vi "DS1820TEMP 3.vi"() -> ()   [LabVIEW 2017]
uses:
  <vilib>/Instr/_visa.llb/VISA Configure Serial Port (Instr).vi
panel:
  in  "stop":bool
  in  "Lim_inf":dbl
  in  "Lim_sup":dbl
  out "WAVE TEMP":dbl(graph)
  out "TEMP GAUGE":dbl(slide) scale=0.0..100.0
  out "TEMP":string
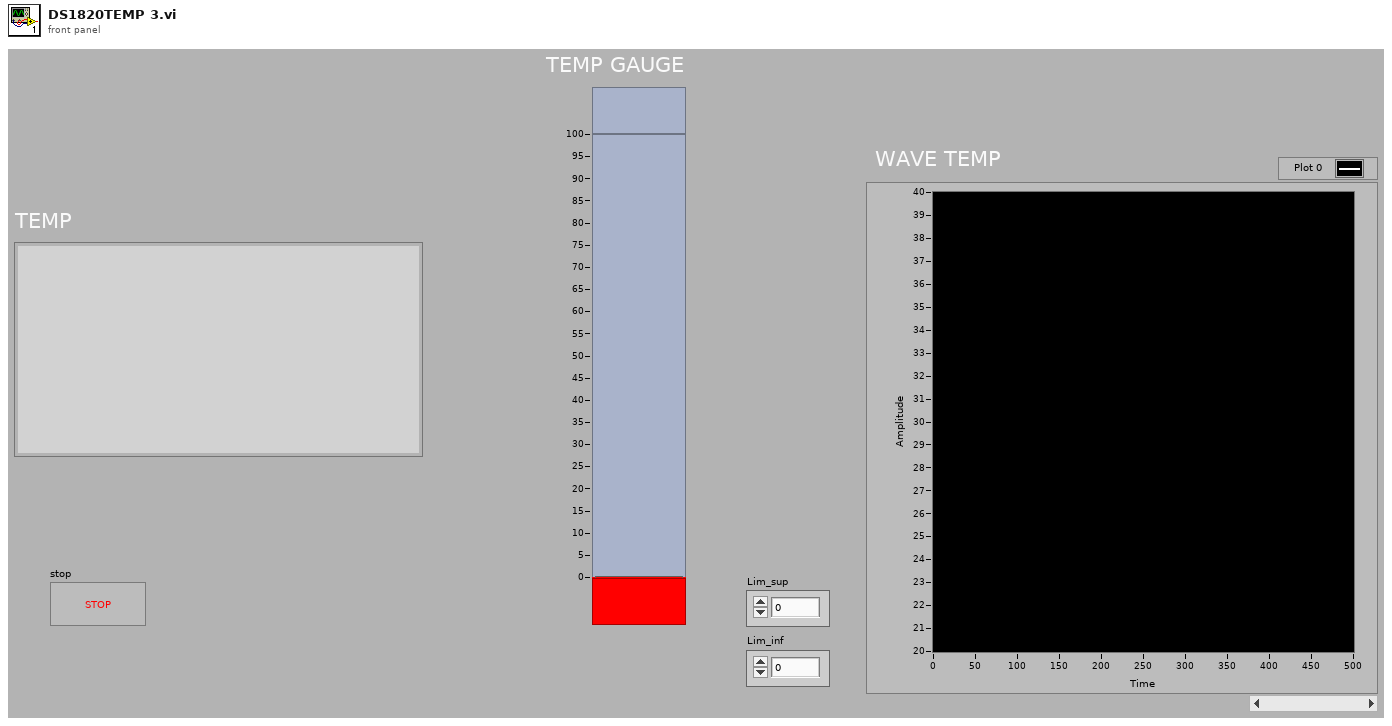
[diagram p1: front panel]
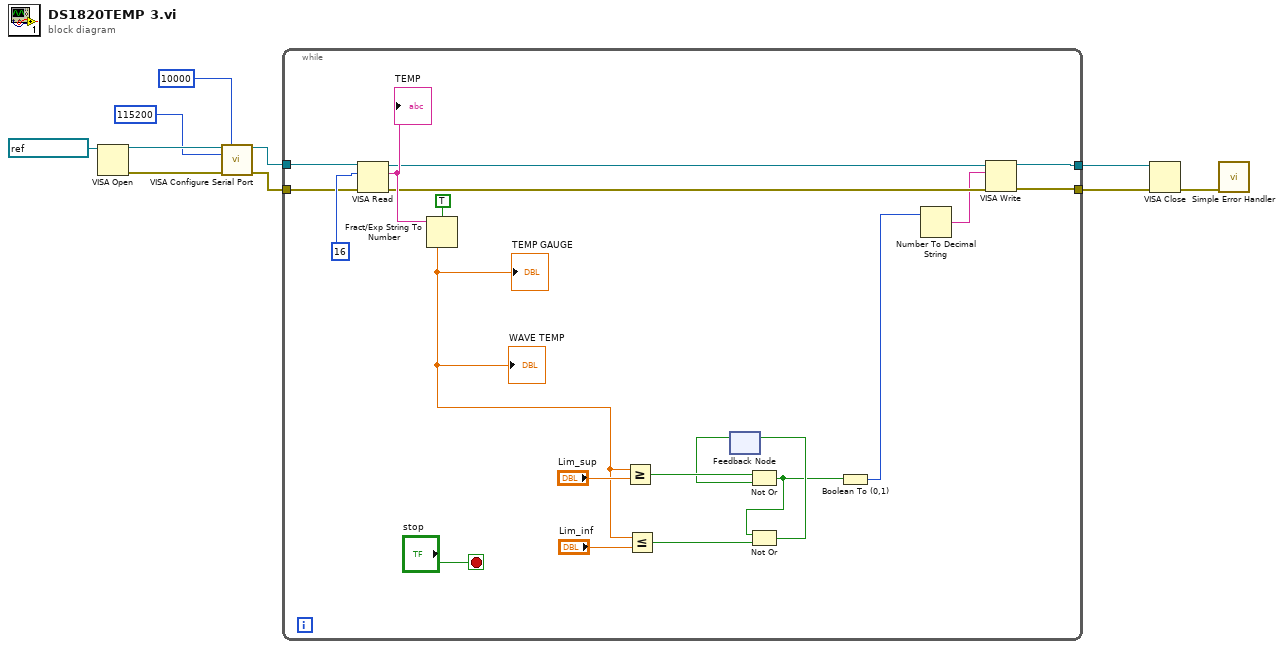
[diagram p0: block diagram]
diagram:
  n1 = VISA Open(VISA resource name=refnum<visa-resource-name> "COM3") -> (VISA resource name=w6:refnum<visa-resource-name>, error out=w5:errorcluster)  [unwired: 4 in]
  n2 = call-poly "VISA Configure Serial Port"("VISA resource name"=w6, "timeout (10sec)"=u32 10000, "baud rate (9600)"=u32 115200, "error in (no error)"=w5) -> ("VISA resource name out"=w8:refnum<visa-resource-name>, "error out"=w7:errorcluster)  [unwired: 10 in]
  n3 = while {
    tunnel: [w15] -> w10
    tunnel: [w14] -> w9
    tunnel: w8 -> [w19]
    tunnel: w7 -> [w18]
    stop <- "stop" stop-if-true
    n4 = VISA Read(VISA resource name=w19, byte count=u32 16, error in (no error)=w18) -> (VISA resource name out=w17:refnum<visa-resource-name>, read buffer=w30:string, error out=w16:errorcluster)  [unwired: 1 out]
    "TEMP" <- w30
    n5 = Fract/Exp String To Number(use system decimal point (T)=TRUE, string=w30) -> (number=w22:dbl)  [unwired: 2 in, 1 out]
    "TEMP GAUGE" <- w22
    "WAVE TEMP" <- w22
    n6 = Greater Or Equal?(x=w22, y="Lim_sup") -> (x >= y?=w27:bool)
    n7 = Less Or Equal?(x=w22, y="Lim_inf") -> (x <= y?=w28:bool)
    n8 = feedback #1() -> (w26:bool)  [unwired: 1 in]
    n9 = Not Or(1:w26, 2:w27) -> (0:w21:bool)
    n10 = Not Or(1:w28, 2:w21) -> (0:w25:bool)
    n11 = feedback-in #1(w25) -> ()
    n12 = Boolean To (0,1)(Boolean=w21) -> (0, 1=w13:i16)
    n13 = Number To Decimal String(number=w13) -> (decimal integer string=w12:string)  [unwired: 1 in]
    n14 = VISA Write(VISA resource name=w17, write buffer=w12, error in (no error)=w16) -> (VISA resource name out=w15:refnum<visa-resource-name>, error out=w14:errorcluster)  [unwired: 1 out]
  }
  n15 = VISA Close(VISA resource name=w10, error in (no error)=w9) -> (error out=w1:errorcluster)
  n16 = call <vilib>:"Simple Error Handler.vi"("error in (no error)"=w1) -> ()  [unwired: 4 in, 5 out]
